vi "TFTP Put File.vi"(5 "net address":string, 6 "Binary (T)":bool=TRUE, 7 "timeout ms (1000)":i32=1000, 8 "error in (no error)":errorcluster, 9 "local path":path, 10 "remote path":string, 11 "Host":string) -> (0 "error out":errorcluster, 2 "file error":errorcluster)   [LabVIEW 8.6]
doc: "Connects to an TFTP server and copies the contents of a single file from the local machine."
panel:
  out "File Size":i64
  out "local port":u16
  out "server port":u16
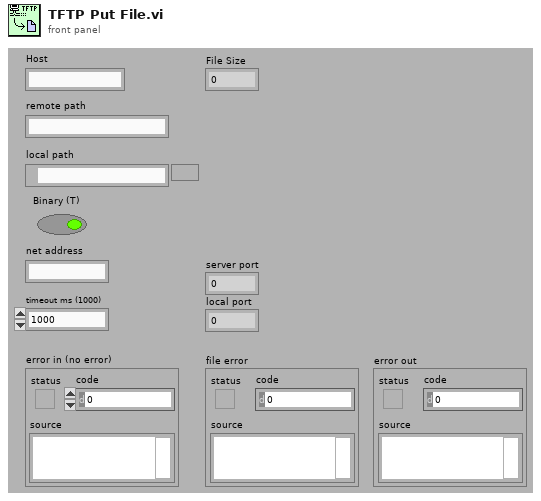
[diagram p1: front panel]
types:
  T1 = enum16{"open", "replace", "create", "open or create", "replace or create", "replace or create with confirmation"}
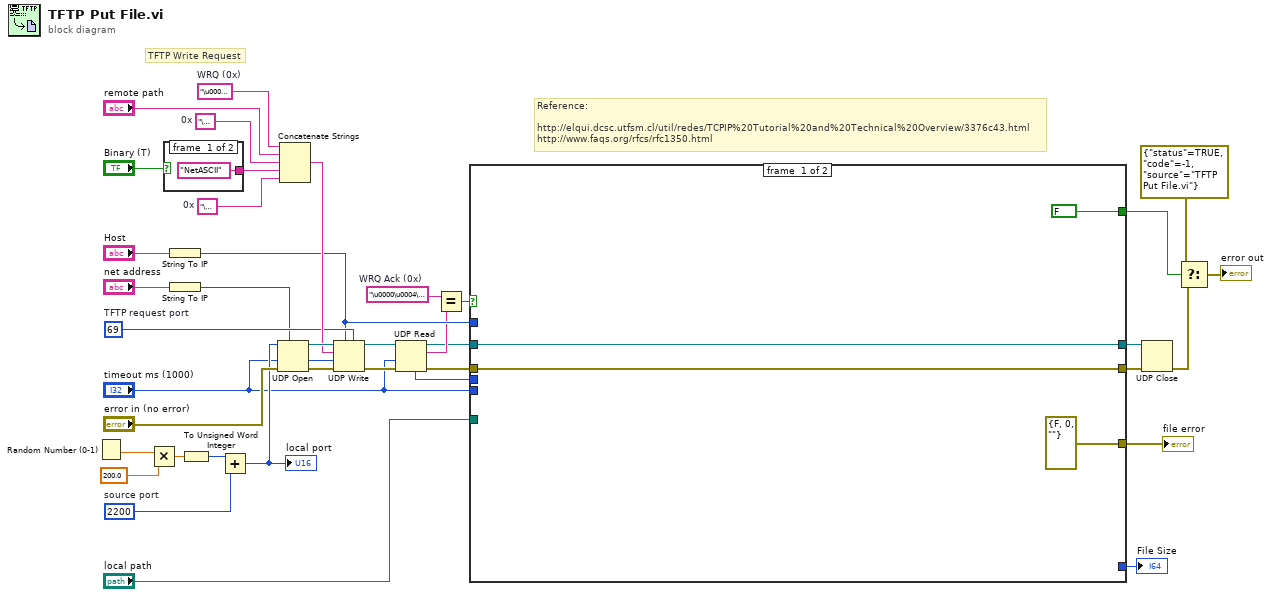
[diagram p0: block diagram]
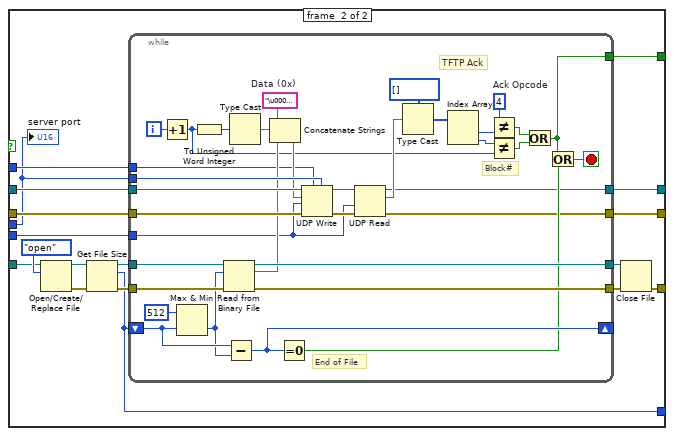
[diagram p2: hidden frame]
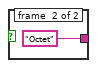
[diagram p3: hidden frame]
diagram:
  w14 = "\u0000\u0004\u0000\u0000"  # WRQ Ack (0x)
  w21 = u16 2200  # source port
  w31 = "\u0000"  # 0x
  w33 = "\u0000"  # 0x
  w35 = "\u0000\u0002"  # WRQ (0x)
  w27 = u16 69  # TFTP request port
  # "Reference:\n\nhttp://elqui.dcsc.utfsm.cl/util/redes/TCPIP%20Tutorial%20and%20Technical%20Overview/3376c43.html\nhttp://www.faqs.org/rfcs/rfc1350.html"
  # "TFTP Write Request"
  n1 = Random Number (0-1)() -> (number: 0 to 1=w23:dbl)
  n2 = Multiply(x=w23, y=200.0) -> (x*y=w25:dbl)
  n3 = case shown="False" "Binary (T)" {
    tunnel: ["NetASCII" "Octet"] -> w32
    frame #0 {
    }
    frame #1 {
    }
  }
  n4 = String To IP(1:"Host") -> (0:w26:u32)
  n5 = String To IP(1:"net address") -> (0:w1:u32)
  n6 = To Unsigned Word Integer(number=w25) -> (unsigned 16bit integer=w22:u16)
  n7 = Add(x=w22, y=w21) -> (x+y=w20:u16)
  "local port" <- w20
  n8 = UDP Open(7:w1, 8:"error in (no error)", 9:"timeout ms (1000)", 11:w20) -> (port=w38:refnum<k16>, 0:w37:errorcluster)  [unwired: 2 out]
  n9 = Concatenate Strings(w35, "remote path", w33, w32, w31) -> (w30:string)
  n10 = UDP Write(address=w26, port or service name=w27, connection ID=w38, data in=w30, 8:w37, 9:"timeout ms (1000)") -> (error out=w18:errorcluster, 3:w17:refnum<k16>)
  n11 = UDP Read(connection ID=w17, timeout ms (25000)="timeout ms (1000)", 8:w18) -> (data out=w15:string, error out=w11:errorcluster, 3:w12:refnum<k16>, 4:w10:u16)  [unwired: 2 out]
  n12 = Equal?(x=w14, y=w15) -> (x = y?=w13:bool)
  n13 = case shown="False" w13 {
    tunnel: w26 -> [_ w63]
    tunnel: [FALSE w59] -> w6
    tunnel: [errorcluster {"status"=FALSE, "code"=0, "source"=""} ("error out") w58] -> w7
    tunnel: "local path" -> [_ w57]
    tunnel: "timeout ms (1000)" -> [_ w56]
    tunnel: w12 -> [w45 w55]
    tunnel: w11 -> [w44 w54]
    tunnel: w10 -> [_ w49]
    tunnel: [w44 w48] -> w9
    tunnel: [w45 w47] -> w8
    tunnel: [_ w46] -> w2
    frame #0 {
    }
    frame #1 {
      n14 = Open/Create/Replace File(file path (use dialog)=w57, operation (0:open)=T1."open") -> (refnum out=w52:refnum<file>, error out=w53:errorcluster)  [unwired: 1 in, 4 out]
      n15 = Get File Size(file=w52, error in=w53) -> (refnum out=w50:refnum<file>, size (in bytes)=w46:i64, 0:w51:errorcluster)
      n16 = while {
        tunnel: w55 -> [w98]
        tunnel: w54 -> [w97]
        tunnel: w63 -> [w64]
        tunnel: w56 -> [w70]
        tunnel: [w87] -> w62
        tunnel: [w86] -> w61
        tunnel: [w85] -> w59
        tunnel: w49 -> [w84]
        shift-right: [w79] -> _
        shift-left: w46 -> [w81]
        tunnel: w51 -> [w82]
        tunnel: w50 -> [w78]
        tunnel: [w66] -> w48
        tunnel: [w65] -> w47
        i -> [w92]
        stop <- w89 stop-if-true
        w73 = "\u0000\u0003"  # Data (0x)
        w93 = u16 4  # Ack Opcode
        # "End of File"
        # "Block#"
        # "TFTP Ack"
        n17 = Increment(x=w92) -> (x+1=w68:i32)
        n18 = Max & Min(x=i64 512 ("count (1)"), y=w81) -> (min(x,y)=w80:i64)  [unwired: 1 out]
        n19 = To Unsigned Word Integer(number=w68) -> (unsigned 16bit integer=w75:u16)
        n20 = Read from Binary File(8:w82, 10:w80, 11:w78) -> (0:w86:errorcluster, 2:w71:string, 3:w87:refnum<file>)  [unwired: 4 out]
        n21 = Subtract(x=w81, y=w80) -> (x-y=w79:i64)
        n22 = Type Cast(x=w75) -> (*(type *) &x=w72:string)  [unwired: 1 out]
        n23 = Concatenate Strings(w73, w72, w71) -> (w74:string)
        n24 = Equal To 0?(x=w79) -> (x = 0?=w67:bool)
        n25 = UDP Write(address=w64, port or service name=w84, connection ID=w98, data in=w74, 8:w97, 9:w70) -> (error out=w76:errorcluster, 3:w77:refnum<k16>)
        n26 = UDP Read(connection ID=w77, timeout ms (25000)=w70, 8:w76) -> (data out=w69:string, error out=w66:errorcluster, 3:w65:refnum<k16>)  [unwired: 3 out]
        n27 = Type Cast(type=u16[] [], x=w69) -> (*(type *) &x=w95:u16[])
        n28 = Index Array(array=w95) -> (element #1=w94:u16, element #2=w88:u16)  [unwired: 2 in]
        n29 = Not Equal?(x=w93, y=w94) -> (x != y?=w90:bool)
        n30 = Not Equal?(x=w88, y=w68) -> (x != y?=w91:bool)
        n31 = Or(x=w90, y=w91) -> (x .or. y?=w85:bool)
        n32 = Or(x=w85, y=w67) -> (x .or. y?=w89:bool)
      }
      n33 = Close File(refnum=w62, error in=w61) -> (error out=w58:errorcluster)  [unwired: 1 out]
      "server port" <- w49
    }
  }
  "file error" <- w7
  "File Size" <- w2
  n34 = UDP Close(connection ID=w8, 8:w9) -> (error out=w5:errorcluster)  [unwired: 1 out]
  n35 = Select(t=errorcluster {"status"=TRUE, "code"=-1, "source"="TFTP Put File.vi"}, s=w6, f=w5) -> (s? t:f=→"error out":errorcluster)
